vi "test_RS-xxx Protocol Factory.vi"(8 "error in (no error)":errorcluster, 11 "TestCase in":refnum<class "Instrument Addon Scripting API Protocol Factories Unit Tests.lvclass">) -> (0 "error out":errorcluster, 3 "TestCase out":refnum<class "Instrument Addon Scripting API Protocol Factories Unit Tests.lvclass">)   [LabVIEW 2023, in "Instrument Addon Scripting API Protocol Factories Unit Tests.lvclass"]
uses:
  Instrument Addon Scripting API Protocol Factories Unit Tests.lvclass
  <vilib>/addons/_JKI Toolkits/VI Tester/TestCase.llb/TestCase.lvclass
  RS-xxx/RS-xxx.lvclass
  RS-xxx/RS-xxx Settings.ctl
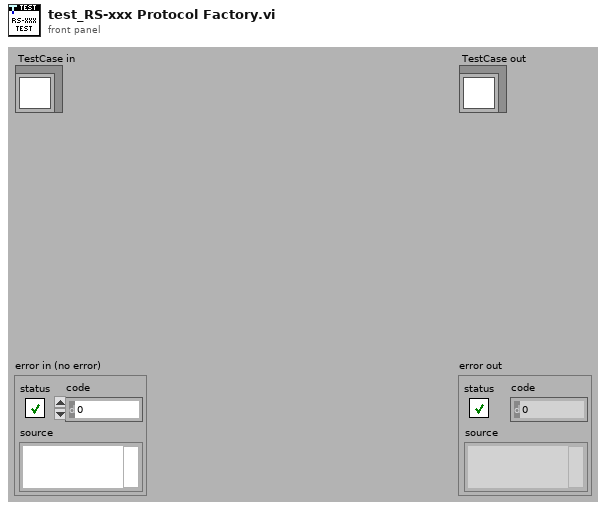
[diagram p1: front panel]
types:
  T1 = typedef "Protocols.lvlib/RS-xxx.lvclass/RS-xxx Settings.ctl" = cluster{"Port":string, "Baud Rate":u32, "Data Bits":u16, "Parity":enum16{"None", "Odd", "Even", "Mark", "Space"}, "Stop Bits":u16, "Flow Control":u16, "XON":enum16{"NUL", "SOH", "STX", "ETX", "EOT", "ENQ", "ACK", "BEL", "BS", "HT", "LF", "VT", "FF", "CR", "SO", "SI", "DLE", "DC1", "DC2", "DC3", "DC4", "NAK", "SYN", "ETB", "CAN", "EM", "SUB", "ESC", "FS", "GS", "RS", "US", "SP", "!", "\"", "#", "$", "%", "&", "'", "(", ")", "*", "+", ",", "- (-)", ".", "/", "0", "1", "2", "3", "4", "5", "6", "7", "8", "9", ":", ";", "<", "=", ">", "?", "@", "A", "B", "C", "D", "E", "F", "G", "H", "I", "J", "K", "L", "M", "N", "O", "P", "Q", "R", "S", "T", "U", "V", "W", "X", "Y", "Z", "[", "\\", "]", "^", "_", "`", "a", "b", "c", "d", "e", "f", "g", "h", "i", "j", "k", "l", "m", "n", "o", "p", "q", "r", "s", "t", "u", "v", "w", "x", "y", "z", "{", "|", "}", "~"}, "XOFF":enum16{"NUL", "SOH", "STX", "ETX", "EOT", "ENQ", "ACK", "BEL", "BS", "HT", "LF", "VT", "FF", "CR", "SO", "SI", "DLE", "DC1", "DC2", "DC3", "DC4", "NAK", "SYN", "ETB", "CAN", "EM", "SUB", "ESC", "FS", "GS", "RS", "US", "SP", "!", "\"", "#", "$", "%", "&", "'", "(", ")", "*", "+", ",", "- (-)", ".", "/", "0", "1", "2", "3", "4", "5", "6", "7", "8", "9", ":", ";", "<", "=", ">", "?", "@", "A", "B", "C", "D", "E", "F", "G", "H", "I", "J", "K", "L", "M", "N", "O", "P", "Q", "R", "S", "T", "U", "V", "W", "X", "Y", "Z", "[", "\\", "]", "^", "_", "`", "a", "b", "c", "d", "e", "f", "g", "h", "i", "j", "k", "l", "m", "n", "o", "p", "q", "r", "s", "t", "u", "v", "w", "x", "y", "z", "{", "|", "}", "~"}, "End Read on Termination Character":bool, "End Write on Termination Character":bool, "Termination Character":u8, "4wireMode":bool, "AssertDTR":bool, "WireMode":i16}
  T2 = cluster{"Port":string, "Baud Rate":u32, "Data Bits":u16, "Parity":enum16{"None", "Odd", "Even", "Mark", "Space"}, "Stop Bits":u16, "Flow Control":u16, "XON":enum16{"NUL", "SOH", "STX", "ETX", "EOT", "ENQ", "ACK", "BEL", "BS", "HT", "LF", "VT", "FF", "CR", "SO", "SI", "DLE", "DC1", "DC2", "DC3", "DC4", "NAK", "SYN", "ETB", "CAN", "EM", "SUB", "ESC", "FS", "GS", "RS", "US", "SP", "!", "\"", "#", "$", "%", "&", "'", "(", ")", "*", "+", ",", "- (-)", ".", "/", "0", "1", "2", "3", "4", "5", "6", "7", "8", "9", ":", ";", "<", "=", ">", "?", "@", "A", "B", "C", "D", "E", "F", "G", "H", "I", "J", "K", "L", "M", "N", "O", "P", "Q", "R", "S", "T", "U", "V", "W", "X", "Y", "Z", "[", "\\", "]", "^", "_", "`", "a", "b", "c", "d", "e", "f", "g", "h", "i", "j", "k", "l", "m", "n", "o", "p", "q", "r", "s", "t", "u", "v", "w", "x", "y", "z", "{", "|", "}", "~"}, "XOFF":enum16{"NUL", "SOH", "STX", "ETX", "EOT", "ENQ", "ACK", "BEL", "BS", "HT", "LF", "VT", "FF", "CR", "SO", "SI", "DLE", "DC1", "DC2", "DC3", "DC4", "NAK", "SYN", "ETB", "CAN", "EM", "SUB", "ESC", "FS", "GS", "RS", "US", "SP", "!", "\"", "#", "$", "%", "&", "'", "(", ")", "*", "+", ",", "- (-)", ".", "/", "0", "1", "2", "3", "4", "5", "6", "7", "8", "9", ":", ";", "<", "=", ">", "?", "@", "A", "B", "C", "D", "E", "F", "G", "H", "I", "J", "K", "L", "M", "N", "O", "P", "Q", "R", "S", "T", "U", "V", "W", "X", "Y", "Z", "[", "\\", "]", "^", "_", "`", "a", "b", "c", "d", "e", "f", "g", "h", "i", "j", "k", "l", "m", "n", "o", "p", "q", "r", "s", "t", "u", "v", "w", "x", "y", "z", "{", "|", "}", "~"}, "End Read on Termination Character":bool, "End Write on Termination Character":bool, "Termination Character":u8, "4wireMode":bool, "AssertDTR":bool, "WireMode":i16}
  T3 = enum16{"NUL", "SOH", "STX", "ETX", "EOT", "ENQ", "ACK", "BEL", "BS", "HT", "LF", "VT", "FF", "CR", "SO", "SI", "DLE", "DC1", "DC2", "DC3", "DC4", "NAK", "SYN", "ETB", "CAN", "EM", "SUB", "ESC", "FS", "GS", "RS", "US", "SP", "!", "\"", "#", "$", "%", "&", "'", "(", ")", "*", "+", ",", "- (-)", ".", "/", "0", "1", "2", "3", "4", "5", "6", "7", "8", "9", ":", ";", "<", "=", ">", "?", "@", "A", "B", "C", "D", "E", "F", "G", "H", "I", "J", "K", "L", "M", "N", "O", "P", "Q", "R", "S", "T", "U", "V", "W", "X", "Y", "Z", "[", "\\", "]", "^", "_", "`", "a", "b", "c", "d", "e", "f", "g", "h", "i", "j", "k", "l", "m", "n", "o", "p", "q", "r", "s", "t", "u", "v", "w", "x", "y", "z", "{", "|", "}", "~"}
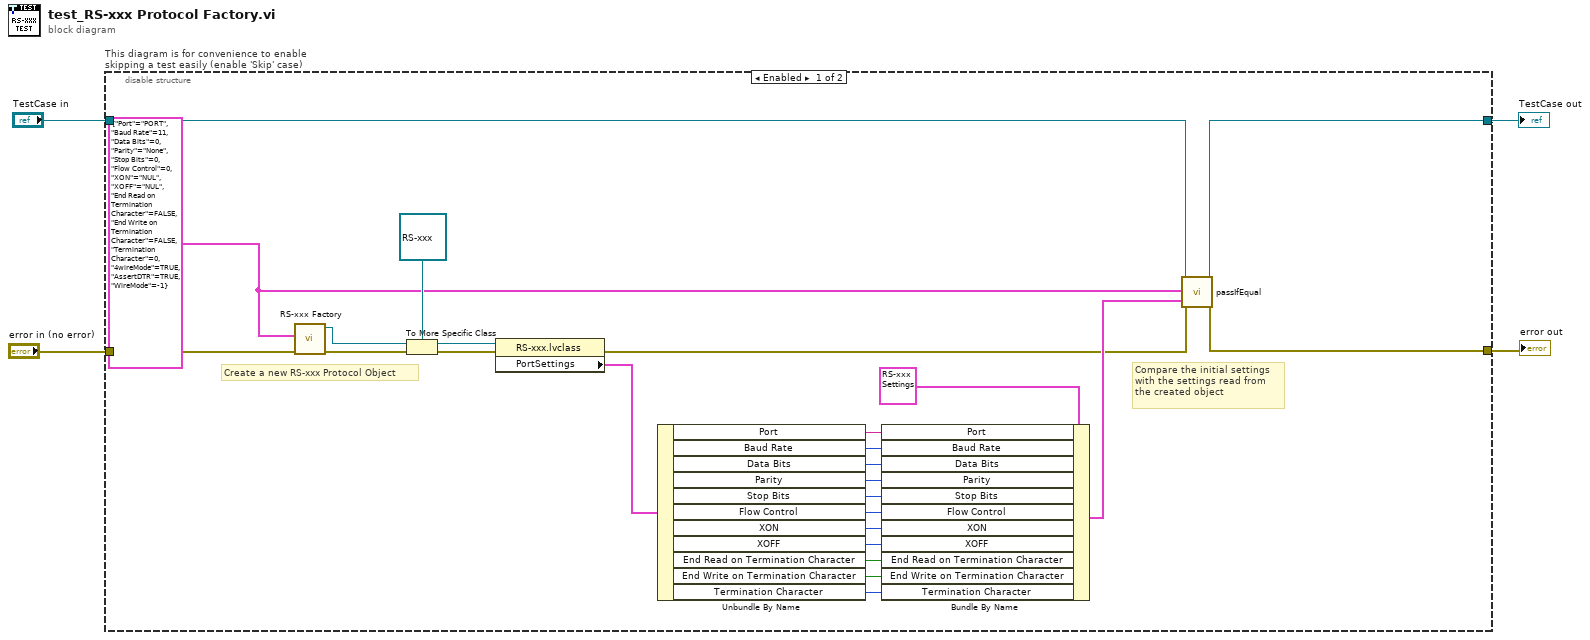
[diagram p0: block diagram]
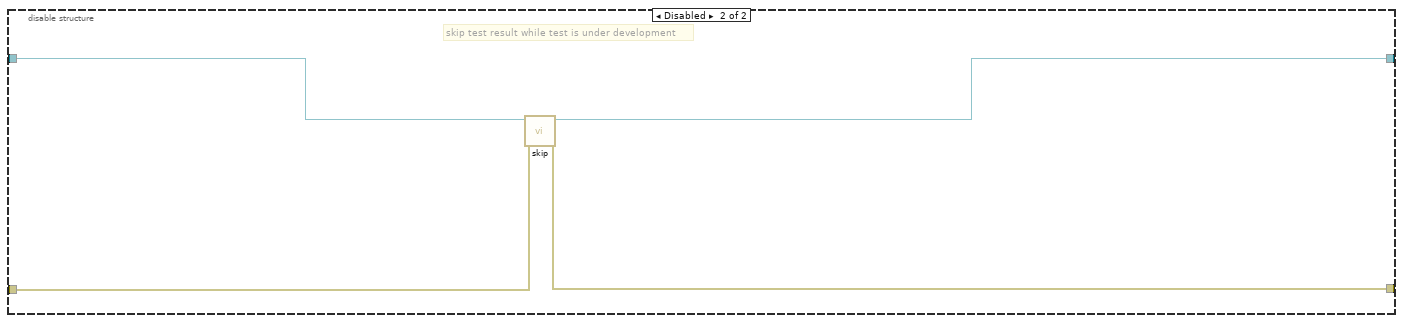
[diagram p2: hidden frame]
diagram:
  n1 = disable-structure "This diagram is for convenience to enable skipping a test easily (enable 'Skip' case)" shown="Enabled" {
    disable-tunnel: "TestCase in" -> [w29 w33]
    disable-tunnel: [w28 w31] -> w1
    disable-tunnel: [w27 w32] -> w3
    disable-tunnel: "error in (no error)" -> [w26 w30]
    frame Enabled {
      w5 = T1 {"Port"="PORT", "Baud Rate"=11, "Data Bits"=0, "Parity"=enum."None", "Stop Bits"=0, "Flow Control"=0, "XON"=enum."NUL", "XOFF"=enum."NUL", "End Read on Termination Character"=FALSE, "End Write on Termination Character"=FALSE, "Termination Character"=0, "4wireMode"=TRUE, "AssertDTR"=TRUE, "WireMode"=-1} ("RS-xxx settings")
      # "Compare the initial settings \nwith the settings read from \nthe created object"
      # "Create a new RS-xxx Protocol Object"
      n2 = call "RS-xxx Factory.vi"("error in (no error)"=w26, "RS-xxx settings"=w5) -> ("error out"=w19:errorcluster, "protocol out"=w18:refnum<class "Protocol Parent.lvclass">)  [unwired: 8 in]
      n3 = To More Specific Class(target class=refnum<class "RS-xxx.lvclass"> refnum ("Protocols.lvlib:RS-xxx.lvclass"), reference=w18, error in=w19) -> (specific class reference=w21:refnum<class "RS-xxx.lvclass">, error out=w20:errorcluster)
      n4 = property class="RS-xxx.lvclass"(reference=w21, error in=w20) -> (error out=w23:errorcluster, "PortSettings"=w22:T2)  [unwired: 1 out]
      n5 = Unbundle By Name(w22) -> ("Port"=w16:string, "Baud Rate"=w15:u32, "Data Bits"=w14:u16, "Parity"=w13:enum16{"None", "Odd", "Even", "Mark", "Space"}, "Stop Bits"=w12:u16, "Flow Control"=w11:u16, "XON"=w10:T3, "XOFF"=w9:T3, "End Read on Termination Character"=w8:bool, "End Write on Termination Character"=w7:bool, "Termination Character"=w6:u8)
      n6 = Bundle By Name(cluster=T1 {"Port"="", "Baud Rate"=0, "Data Bits"=0, "Parity"=enum."None", "Stop Bits"=0, "Flow Control"=0, "XON"=enum."NUL", "XOFF"=enum."NUL", "End Read on Termination Character"=FALSE, "End Write on Termination Character"=FALSE, "Termination Character"=0, "4wireMode"=TRUE, "AssertDTR"=TRUE, "WireMode"=-1} ("PortSettings"), "Port"=w16, "Baud Rate"=w15, "Data Bits"=w14, "Parity"=w13, "Stop Bits"=w12, "Flow Control"=w11, "XON"=w10, "XOFF"=w9, "End Read on Termination Character"=w8, "End Write on Termination Character"=w7, "Termination Character"=w6) -> (w24:T1)
      n7 = call-dynamic "passIfEqual.vi"("error in (no error)"=w23, "y"=w24, "x"=w5, "TestCase in"=w29) -> ("error out"=w27:errorcluster, "TestCase out"=w28:refnum<class "Instrument Addon Scripting API Protocol Factories Unit Tests.lvclass">)  [unwired: 6 in]
    }
    frame Disabled {
      # "skip test result while test is under development"
      n8 = call <vilib>:"skip.vi"("error in (no error)"=w30, "TestCase in"=w33) -> ("error out"=w32:errorcluster, "TestCase out"=w31:refnum<class "Instrument Addon Scripting API Protocol Factories Unit Tests.lvclass">)  [unwired: 8 in]
    }
  }
  "error out" <- w3
  "TestCase out" <- w1
